vi "ConfigStdWFCh1.vi"(0 "object in":refnum<class "AFG3022B.lvclass">, 2 "Configdatastd":T1, 5 "error in (no error)":errorcluster) -> (14 "object out":refnum<class "AFG3022B.lvclass">, 19 "error out":errorcluster)   [LabVIEW 2019, in "AFG3022B.lvclass"]
uses:
  AFG3022B.lvclass
  AFG3022B.lvclass/AFG3022B.ctl
  Tektronix AFG 3000 Series/Tektronix AFG 3000 Series.lvlib
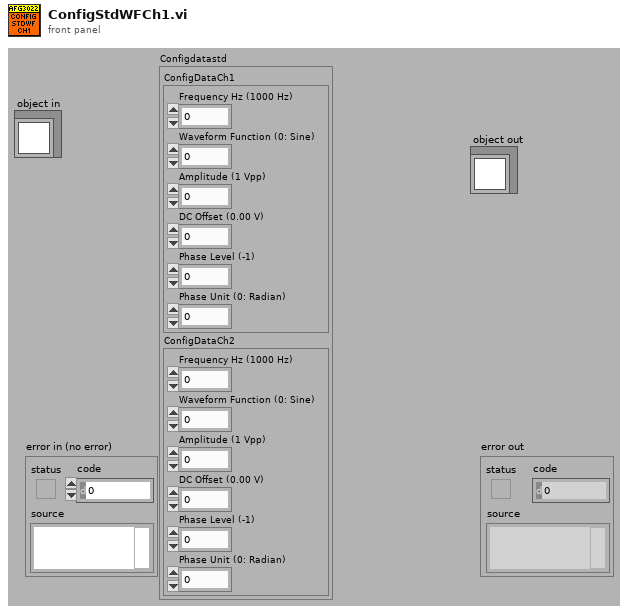
[diagram p1: front panel]
types:
  T1 = cluster{"ConfigDataCh1":cluster{"Frequency Hz (1000 Hz)":dbl, "Waveform Function (0: Sine)":u16, "Amplitude (1 Vpp)":dbl, "DC Offset (0.00 V)":dbl, "Phase Level (-1)":dbl, "Phase Unit (0: Radian)":u16}, "ConfigDataCh2":cluster{"Frequency Hz (1000 Hz)":dbl, "Waveform Function (0: Sine)":u16, "Amplitude (1 Vpp)":dbl, "DC Offset (0.00 V)":dbl, "Phase Level (-1)":dbl, "Phase Unit (0: Radian)":u16}}
  T2 = cluster{"Frequency Hz (1000 Hz)":dbl, "Waveform Function (0: Sine)":u16, "Amplitude (1 Vpp)":dbl, "DC Offset (0.00 V)":dbl, "Phase Level (-1)":dbl, "Phase Unit (0: Radian)":u16}
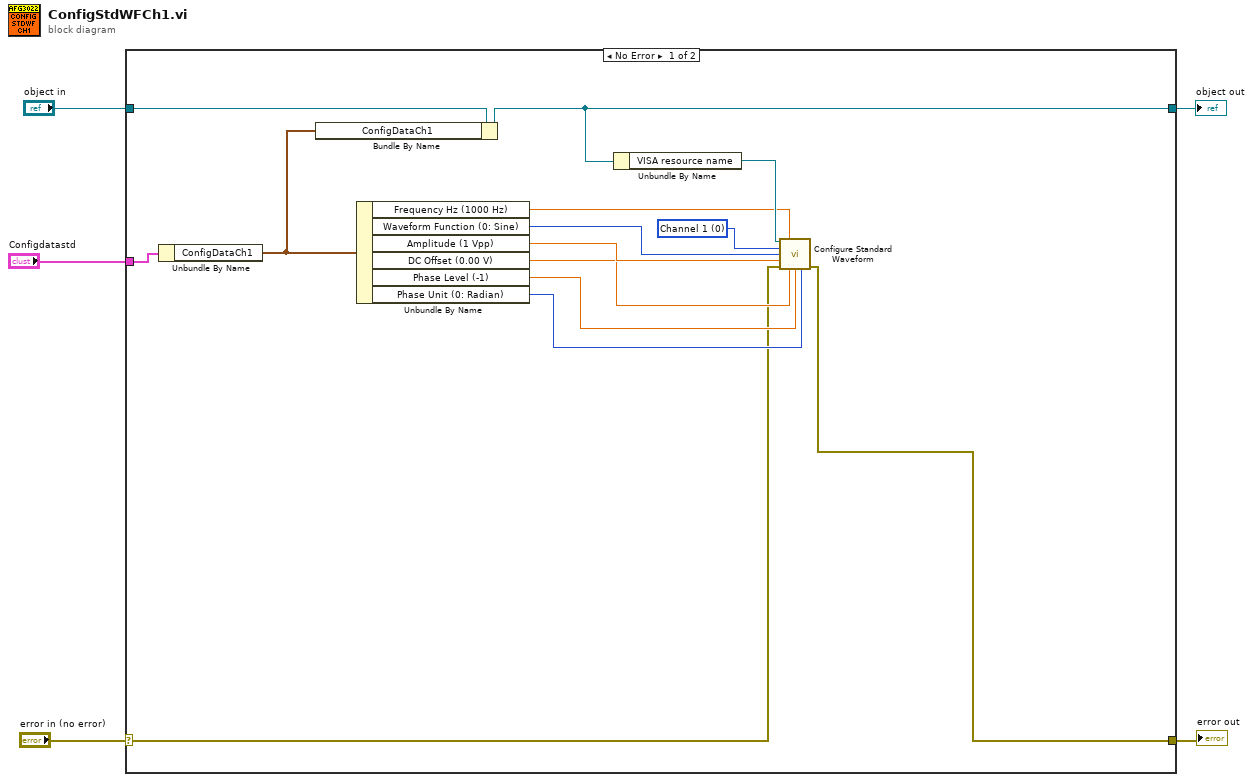
[diagram p0: block diagram]
diagram:
  n1 = case shown="No Error" "error in (no error)" {
    selector: "error in (no error)" -> [w10 w21]
    tunnel: [w7 w21] -> w4
    tunnel: [w11 w20] -> w2
    tunnel: "object in" -> [w19 w20]
    tunnel: "Configdatastd" -> [w8 _]
    frame No Error {
      w9 = u16 0 items=["Channel 1", "Channel 2"] ("Channel (0: Channel 1)")
      n2 = Unbundle By Name(w8) -> ("ConfigDataCh1"=w6:T2)
      n3 = Bundle By Name(cluster=w19, "ConfigDataCh1"=w6) -> (w11:refnum<class "AFG3022B.lvclass">)
      n4 = Unbundle By Name(w6) -> ("Frequency Hz (1000 Hz)"=w17:dbl, "Waveform Function (0: Sine)"=w16:u16, "Amplitude (1 Vpp)"=w15:dbl, "DC Offset (0.00 V)"=w14:dbl, "Phase Level (-1)"=w13:dbl, "Phase Unit (0: Radian)"=w12:u16)
      n5 = Unbundle By Name(w11) -> ("VISA resource name"=w18:refnum<visa-resource-name>)
      n6 = call "Configure Standard Waveform.vi"("VISA resource name"=w18, "Frequency (1000 Hz)"=w17, "Channel (0: Channel 1)"=w9, "Waveform Function (0: Sine)"=w16, "Amplitude (1 Vpp)"=w15, "error in (no error)"=w10, "DC Offset (0.00 V)"=w14, "Phase Level (-1)"=w13, "Phase Unit (0: Radian)"=w12) -> ("error out"=w7:errorcluster)  [unwired: 5 in, 1 out]
    }
    frame Error {
    }
  }
  "error out" <- w4
  "object out" <- w2
